vi "Set Mode.vi"(0 "QCS.lvclass in":refnum<class "QCS.lvclass">, 1 "On&G 0":T1, 2 "On&G 1":T1, 3 "On&G 2":T1, 4 "On&G 3":T1, 5 "error in (no error)":errorcluster) -> (14 "QCS.lvclass out":refnum<class "QCS.lvclass">, 19 "error out":errorcluster)   [LabVIEW 2016, in "QCS.lvclass"]
uses:
  Lib.llb/QCS.lvclass
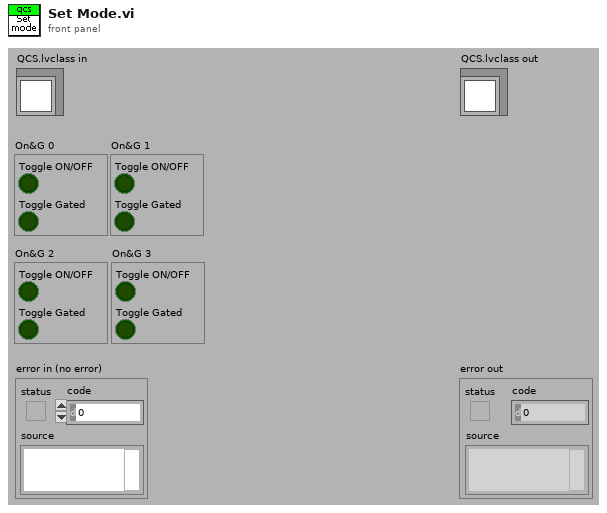
[diagram p1: front panel]
types:
  T1 = cluster{"Toggle ON/OFF":bool, "Toggle Gated":bool}
  T2 = typedef "CS Data.ctl" = cluster{"Range":u8, "Current":dbl, "Current (string)":string, "On?":bool, "G?":bool, "I?":bool, "Err?":bool}
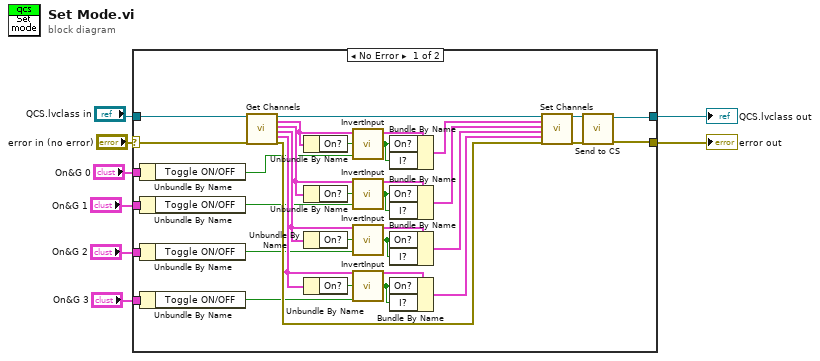
[diagram p0: block diagram]
diagram:
  n1 = case shown="No Error" "error in (no error)" {
    selector: "error in (no error)" -> [w25 w42]
    tunnel: [w13 w42] -> w8
    tunnel: [w14 w41] -> w7
    tunnel: "QCS.lvclass in" -> [w39 w41]
    tunnel: "On&G 3" -> [w24 _]
    tunnel: "On&G 2" -> [w21 _]
    tunnel: "On&G 1" -> [w18 _]
    tunnel: "On&G 0" -> [w17 _]
    frame No Error {
      n2 = Unbundle By Name(w17) -> ("Toggle ON/OFF"=w19:bool)
      n3 = Unbundle By Name(w18) -> ("Toggle ON/OFF"=w20:bool)
      n4 = Unbundle By Name(w21) -> ("Toggle ON/OFF"=w22:bool)
      n5 = Unbundle By Name(w24) -> ("Toggle ON/OFF"=w23:bool)
      n6 = call-dynamic "Get Channels.vi"("CS.lvclass in"=w39, "error in (no error)"=w25) -> ("CS.lvclass out"=w38:refnum<class "QCS.lvclass">, "I0"=w36:T2, "I1"=w30:T2, "I2"=w29:T2, "I3"=w28:T2, "error out"=w40:errorcluster)  [unwired: 12 in]
      n7 = Unbundle By Name(w36) -> ("On?"=w37:bool)
      n8 = Unbundle By Name(w30) -> ("On?"=w34:bool)
      n9 = Unbundle By Name(w29) -> ("On?"=w33:bool)
      n10 = Unbundle By Name(w28) -> ("On?"=w32:bool)
      n11 = call "InvertInput.vi"("In"=w37, "Invert?"=w19) -> ("Out"=w9:bool)
      n12 = call "InvertInput.vi"("In"=w34, "Invert?"=w20) -> ("Out"=w10:bool)
      n13 = call "InvertInput.vi"("In"=w33, "Invert?"=w22) -> ("Out"=w11:bool)
      n14 = call "InvertInput.vi"("In"=w32, "Invert?"=w23) -> ("Out"=w12:bool)
      n15 = Bundle By Name(cluster=w36, "On?"=w9, "I?"=w9) -> (w35:T2)
      n16 = Bundle By Name(cluster=w30, "On?"=w10, "I?"=w10) -> (w31:T2)
      n17 = Bundle By Name(cluster=w29, "On?"=w11, "I?"=w11) -> (w27:T2)
      n18 = Bundle By Name(cluster=w28, "On?"=w12, "I?"=w12) -> (w26:T2)
      n19 = call-dynamic "Set Channels.vi"("CS.lvclass in"=w38, "I0"=w35, "I1"=w31, "I2"=w27, "I3"=w26, "error in (no error)"=w40) -> ("CS.lvclass out"=w16:refnum<class "QCS.lvclass">, "error out"=w15:errorcluster)  [unwired: 12 in]
      n20 = call-dynamic "Send to CS.vi"("error in (no error)"=w15, "QCS in"=w16) -> ("error out"=w13:errorcluster, "QCS out"=w14:refnum<class "QCS.lvclass">)  [unwired: 8 in]
    }
    frame Error {
    }
  }
  "error out" <- w8
  "QCS.lvclass out" <- w7
